vi "ort_fit_start.vi"(8 "inputValid":bool, 10 "ort.fit.p.params":T1, 11 "data":cluster{"index":u16, "data":i16}) -> ()   [LabVIEW 2016]
uses:
  <vilib>/rvi/Emulation/niFpgaSctlEmulationGetInTimedLoop.vi
  <vilib>/rvi/Emulation/niFpgaEmulationIsFPGAContextNoSignature.vi
  <vilib>/rvi/DataTransferAndStorage/Container/Common/niFpgaContainerGetUniqueNameForEmu.vi
  <vilib>/rvi/eio/common/nirviEmuReportErrorAndStop.vi
  <vilib>/rvi/Emulation/niFpgaProcessEmulError.vi
  <vilib>/rvi/DataTransferAndStorage/Container/XNode/niFpgaContainer.xnode
  <vilib>/rvi/DataTransferAndStorage/Handshake/Emulation/niFpgaHandshakeEmulation.vi
  <vilib>/rvi/DataTransferAndStorage/Register/Emulation/niFpgaRegisterEmulation.vi
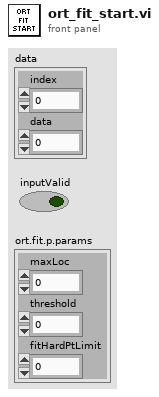
[diagram p1: front panel]
types:
  T1 = cluster{"maxLoc":u16, "threshold":i16, "fitHardPtLimit":u16}
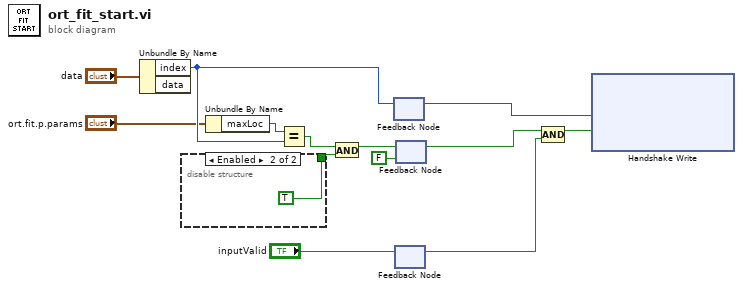
[diagram p0: block diagram]
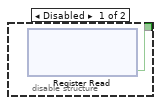
[diagram p2: hidden frame]
diagram:
  n1 = Unbundle By Name("data") -> ("index"=w13:u16)  [unwired: 1 out]
  n2 = disable-structure shown="Enabled" {
    disable-tunnel: [w14 TRUE ("Data")] -> w10
    frame Disabled {
      n3 = xnode "Register Read"() -> ("Data"=w14:bool)  [unwired: 1 in, 1 out]
    }
    frame Enabled {
    }
  }
  n4 = Unbundle By Name("ort.fit.p.params") -> ("maxLoc"=w3:u16)
  n5 = Equal?(x=w3, y=w13) -> (x = y?=w4:bool)
  n6 = And(x=w4, y=w10) -> (x .and. y?=w8:bool)
  n7 = feedback #1() -> (w6:u16)  [unwired: 1 in]
  n8 = feedback-in #1(w13) -> ()
  n9 = feedback-in #2("inputValid") -> ()
  n10 = feedback #2() -> (w1:bool)  [unwired: 1 in]
  n11 = feedback #3(FALSE) -> (w5:bool)
  n12 = feedback-in #3(w8) -> ()
  n13 = Compound Arithmetic op=AND(w5, w1) -> (w9:bool)
  n14 = xnode ("Handshake Write")("Data"=w6, "Input Valid"=w9) -> ()  [unwired: 1 in, 2 out]
